vi "Probability % to compare.vi"(11 "probability %":dbl) -> (3 "probability compare":u16)   [LabVIEW 2020, in "Engine Simulation Toolkit Shared.lvlib"]
uses:
  Engine Simulation Toolkit Shared.lvlib
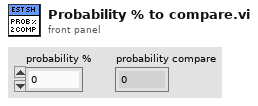
[diagram p1: front panel]
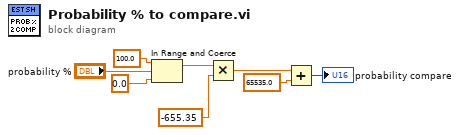
[diagram p0: block diagram]
diagram:
  n1 = In Range and Coerce(upper limit=100.0, x="probability %", lower limit=0.0) -> (coerced(x)=w5:dbl)  [unwired: 1 out]
  n2 = Multiply(x=w5, y=-655.35) -> (x*y=w6:dbl)
  n3 = Add(x=w6, y=65535.0) -> (x+y=→"probability compare":u16)
